vi "Lin_byteLog.vi"(7 "r/w":enum16{"read", "write", "init"}(ring), 10 "RespGood?":string[](array[string]), 11 "TxRx Data":string[][](array[string])) -> (3 "log":string[][](array[string]))   [LabVIEW 2018]
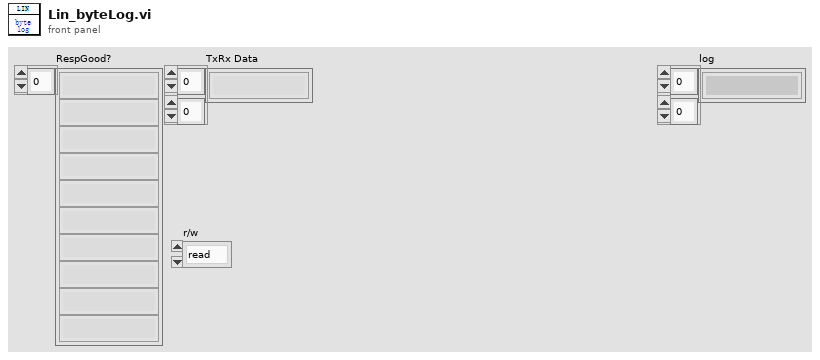
[diagram p1: front panel]
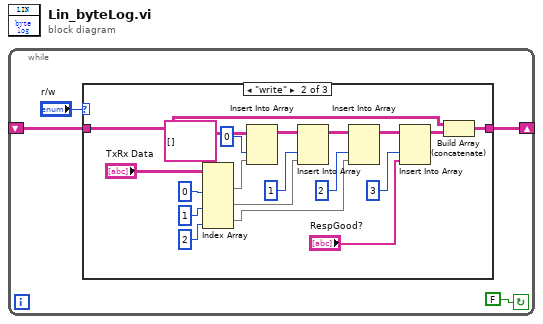
[diagram p0: block diagram]
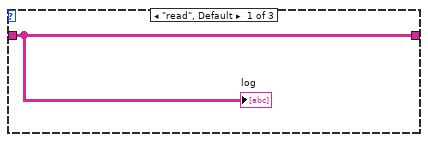
[diagram p2: hidden frame]
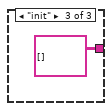
[diagram p3: hidden frame]
diagram:
  n1 = while {
    shift-right: [w1] -> _
    shift-left: _ -> [w3]
    stop <- FALSE continue-if-true
    n2 = case shown="\"write\"" "r/w" {
      tunnel: w3 -> [w5 w9 _]
      tunnel: [w5 w6 string[][] []] -> w1
      frame "read", Default {
        "log" <- w5
      }
      frame "write" {
        n3 = Index Array(array="TxRx Data", index (col) #1=0 ("禁用的索引 (列)"), index (col) #2=1 ("索引 (列)"), index (col) #3=2 ("索引 (列)")) -> (element #1=w14:string[], element #2=w13:string[], element #3=w12:string[])  [unwired: 3 in]
        n4 = Insert Into Array(array=string[][] [] ("数组"), index (col)=0 ("索引 (列)"), new element=w14) -> (w20:string[][])  [unwired: 1 in]
        n5 = Insert Into Array(array=w20, index (col)=1 ("禁用的索引 (列)"), new element=w13) -> (w18:string[][])  [unwired: 1 in]
        n6 = Insert Into Array(array=w18, index (col)=2 ("禁用的索引 (列)"), new element=w12) -> (w16:string[][])  [unwired: 1 in]
        n7 = Insert Into Array(array=w16, index (col)=3 ("禁用的索引 (列)"), new element="RespGood?") -> (w7:string[][])  [unwired: 1 in]
        n8 = Build Array (concatenate)(w9, w7) -> (w6:string[][])
      }
      frame "init" {
      }
    }
  }
